vi "Initiate [TRG] Core.vi"(8 "error in (no error)":errorcluster, 11 "CS++DCPwr in":refnum<class "CS++DCPwr.lvclass">) -> (0 "error out":errorcluster, 3 "CS++DCPwr out":refnum<class "CS++DCPwr.lvclass">)   [LabVIEW 2013, in "CS++DCPwr.lvlib" / "CS++DCPwr.lvclass"]
doc: "This VI initiates output changes that you previously specified. After you call this VI, the power supply waits for the trigger you specify with the IviDCPwr Configure Trigger Source [TRG] VI. After the power supply detects the trigger, it updates its voltage level and current limit to the values you specify with the IviDCPwr Configure Triggered Voltage Level [TRG] and IviDCPwr Configure Triggered Current Limit [TRG] VIs.\n\nNotes:\n\n(1) This VI is part of the IviDCPwrTrigger [TRG] extension group."
uses:
  CS++DCPwr.lvclass
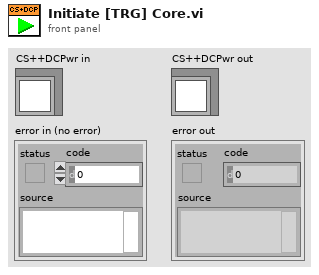
[diagram p1: front panel]
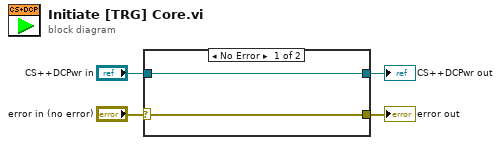
[diagram p0: block diagram]
diagram:
  n1 = case shown="No Error" "error in (no error)" {
    selector: "error in (no error)" -> [w5 w8]
    tunnel: [w5 w8] -> w3
    tunnel: [w6 w7] -> w1
    tunnel: "CS++DCPwr in" -> [w6 w7]
    frame No Error {
    }
    frame Error {
    }
  }
  "error out" <- w3
  "CS++DCPwr out" <- w1
